vi "Get PyObject and Method Names.vi"(8 "error in (no error)":errorcluster, 11 "Node in":refnum<class "PyObject.lvclass">) -> (0 "error out":errorcluster, 1 "Functions":T1(array[cluster]), 2 "Object Name":string, 3 "Node out":refnum<class "PyObject.lvclass">)   [LabVIEW 2020, in "jki_python_bridge.lvlib" / "PyObject.lvclass"]
uses:
  PyObject.lvclass
  PyObject.lvclass/PyObject.ctl
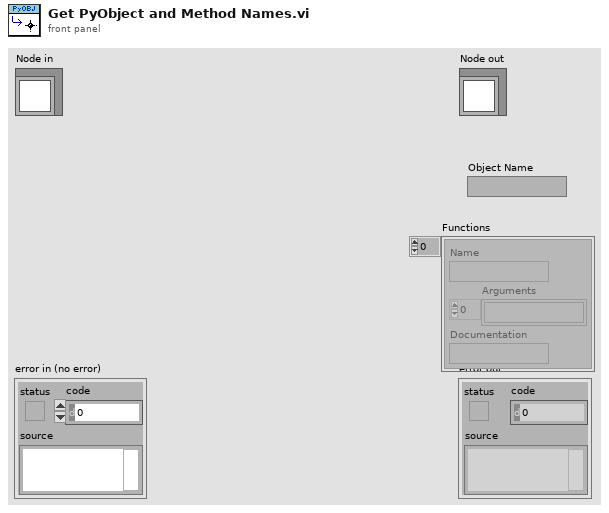
[diagram p1: front panel]
types:
  T1 = cluster{"Name":string, "Arguments":string[], "Documentation":string}[]
  T2 = typedef "jki_python_bridge.lvlib/PyObject.lvclass/Private Data.ctl" = cluster{"Call Registration":T3, "Functions":T4[], "Object Name":string}
  T3 = typedef "jki_python_bridge.lvlib/Server.lvclass/Python Method Call - Event Registration.ctl" = refnum<event-registration>
  T4 = typedef "JKI_Python_Bridge_for_LV.lvlib/PyObject.lvclass/PyObject Method.ctl" = cluster{"Name":string, "Arguments":string[], "Documentation":string}
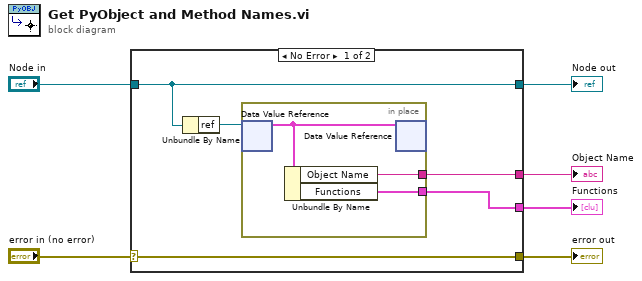
[diagram p0: block diagram]
diagram:
  n1 = case shown="No Error" "error in (no error)" {
    selector: "error in (no error)" -> [w11 w15]
    tunnel: [w11 w15] -> w5
    tunnel: [w10 w16] -> w3
    tunnel: "Node in" -> [w10 w16]
    tunnel: [w8 _] -> w2
    tunnel: [w7 _] -> w1
    frame No Error {
      n2 = Unbundle By Name(w10) -> ("ref"=w9:refnum<data-value>)
      n3 = in-place {
        in-place-border: [w13] -> w8
        in-place-border: [w12] -> w7
        n4 = in-place-dvr #1(w9) -> (w14:T2)  [unwired: 1 out]
        n5 = Unbundle By Name(w14) -> ("Object Name"=w13:string, "Functions"=w12:T4[])
        n6 = in-place-dvr #1(w14) -> ()  [unwired: 2 out]
      }
    }
    frame Error {
    }
  }
  "error out" <- w5
  "Node out" <- w3
  "Object Name" <- w2
  "Functions" <- w1
